vi "Server.vi"(7 "Server Alias":string, 10 "Ports":T2={"KA Port (9007)"=9007, "LtoP Port (9008)"=9008, "PtoL Port (9009)"=9009}, 11 "Local IP Address for LabVIEW Server":string="localhost") -> ()   [LabVIEW 2013, in "TS.lvlib"]
doc: "This VI does the actual TCP/IP connection with the Python side. It has three communication loops: Keep-Alive, LabVIEW-to-Python, and Python-to-LabVIEW. There's also an internal keep-alive loop, where the server has to be \"petted\" every so often, or it shuts down. This server is called dynamically so as to disconnect it from the user's framework."
uses:
  TS.lvlib
  LabVIEW Example/Supporting Code/Script Running.ctl
  LabVIEW Python Connector Message.ctl
  Ports - Keep-Alive, LabVIEW-to-Python, Python-to-LabVIEW.ctl
panel:
  out "PtoL Message":T1={"Command"="zxcvbnm,", "Data"=["asdfghjk", "qwertyui"], "Script ID"=0, "LabVIEW Server ID"="zxcvbnm,", "Python Message ID"=0}
  out "LtoP Iteration Inner":i32
  out "python response":T1={"Command"="zxcvbnm,", "Data"=["asdfghjk", "qwertyui"], "Script ID"=0, "LabVIEW Server ID"="zxcvbnm,", "Python Message ID"=0}
  out "KA Iteration":i32
  out "LtoP Messages":i32
  out "PtoL Messages":i32
  out "KA Timeout":dbl
  out "KA Messages":i32
  out "KA Message":T1={"Command"="", "Data"=[], "Script ID"=0, "LabVIEW Server ID"="zxcvbnm,", "Python Message ID"=0}
  out "LtoP Sent Message":T1={"Command"="zxcvbnm,", "Data"=["asdfghjk", "qwertyui"], "Script ID"=0, "LabVIEW Server ID"="zxcvbnm,", "Python Message ID"=0}
  out "LtoP Iteration Outer":i32
  out "LtoP Last Error":errorcluster
  out "LtoP Last Error Timestamp":timestamp
  out "LtoP length":i32
  out "LtoP Recreating":bool
  out "PtoL Iteration":i32
  out "PtoL Last Error":errorcluster
  out "PtoL Last Error Timestamp":timestamp
  out "PtoL length":i32
  out "PtoL Recreating":bool
  out "Writer Error":errorcluster
  out "Keep-Alive Last Error Timestamp":timestamp
  out "KA length":i32
  out "Keep-Alive Recreating":bool
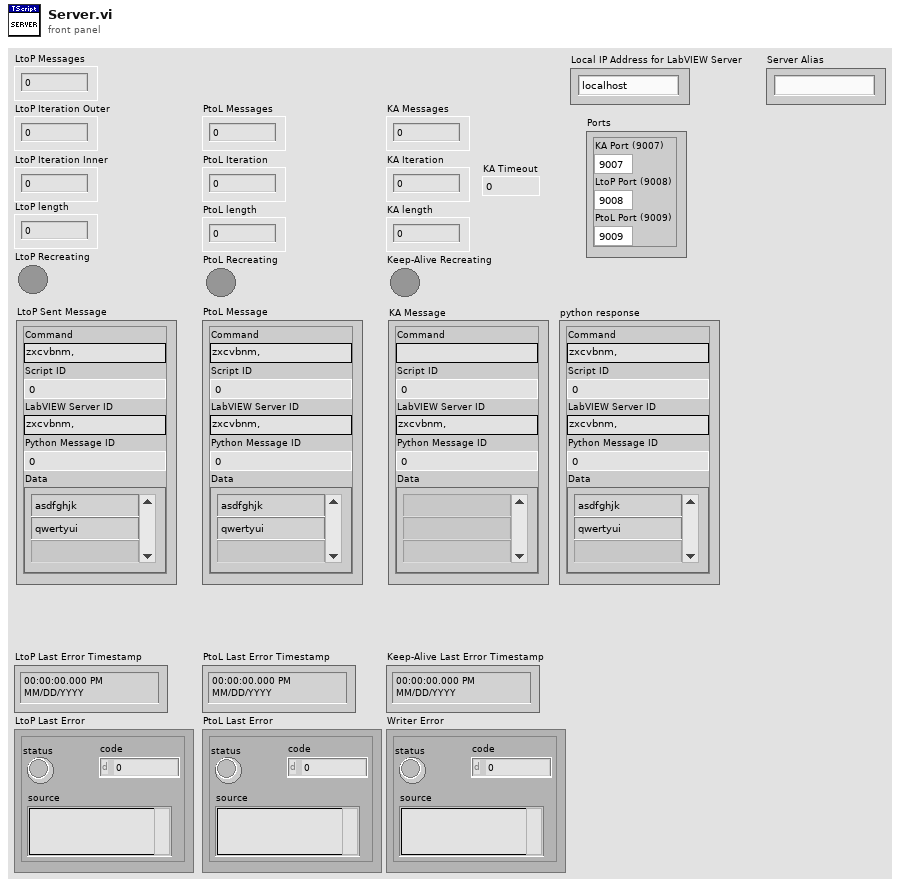
[diagram p1: front panel]
types:
  T1 = typedef "TS.lvlib/LabVIEW Python Connector Message.ctl" = cluster{"Command":string, "Data":string[], "Script ID":i64, "LabVIEW Server ID":string, "Python Message ID":i32}
  T2 = typedef "TS.lvlib/Ports - Keep-Alive, LabVIEW-to-Python, Python-to-LabVIEW.ctl" = cluster{"KA Port (9007)":u16, "LtoP Port (9008)":u16, "PtoL Port (9009)":u16}
  T3 = typedef "TS.lvlib/Script Running.ctl" = cluster{"Script ID":i64, "Script Running?":bool}
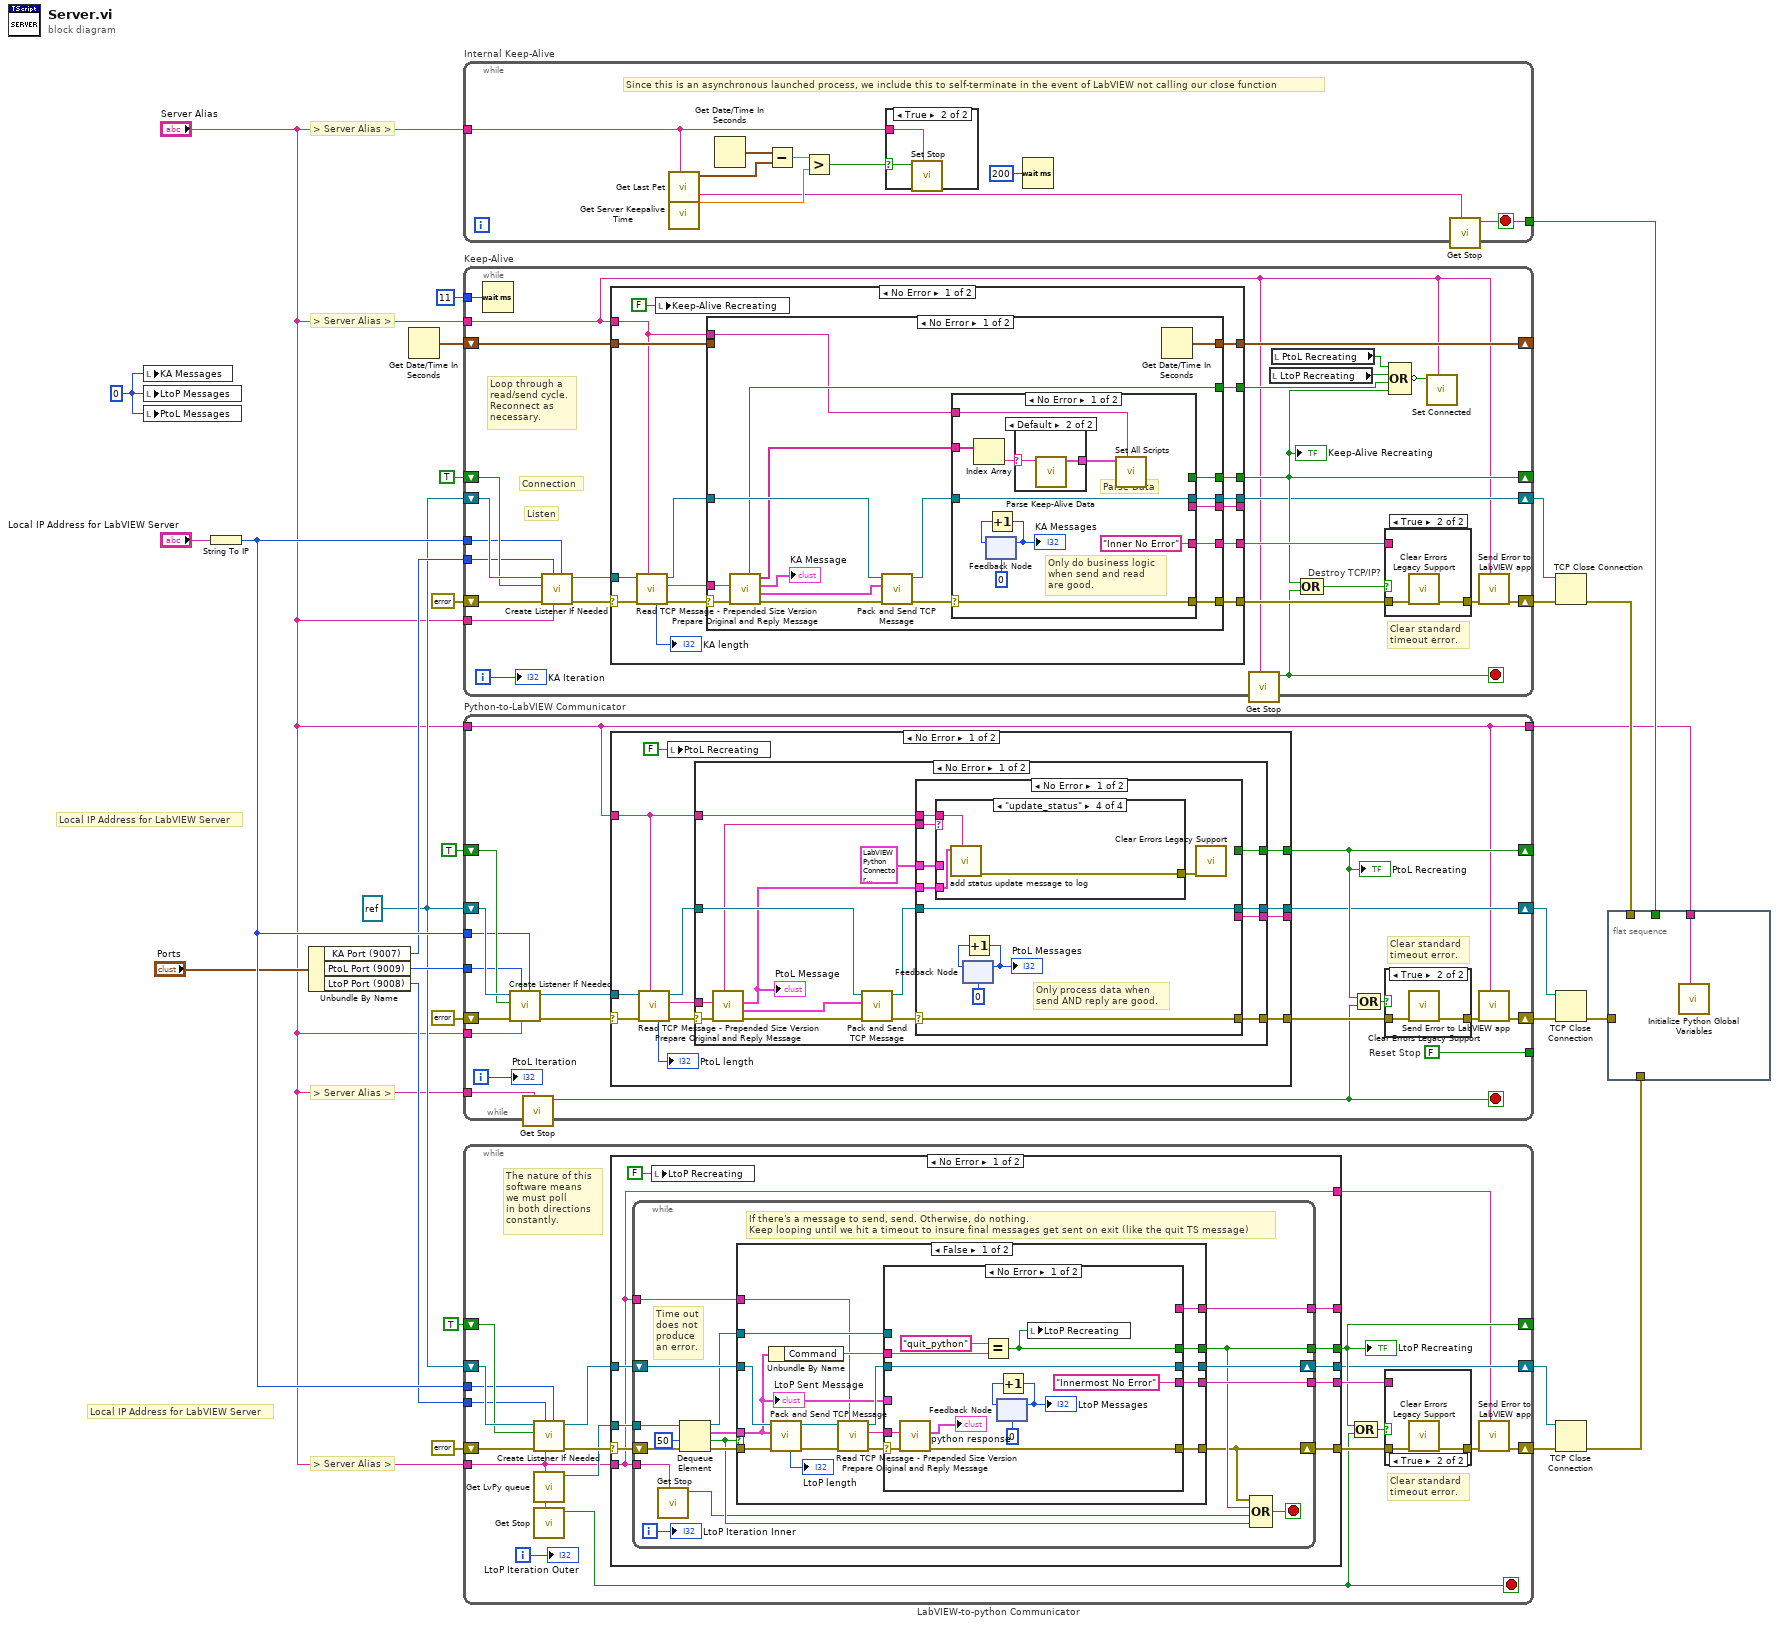
[diagram p0: block diagram]
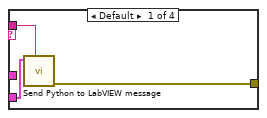
[diagram p2: hidden frame]
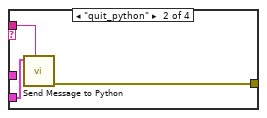
[diagram p3: hidden frame]
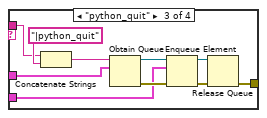
[diagram p4: hidden frame]
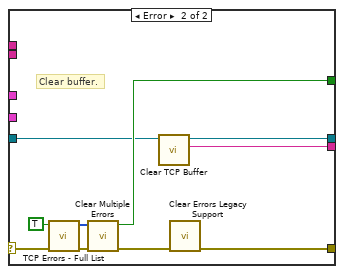
[diagram p5: hidden frame]
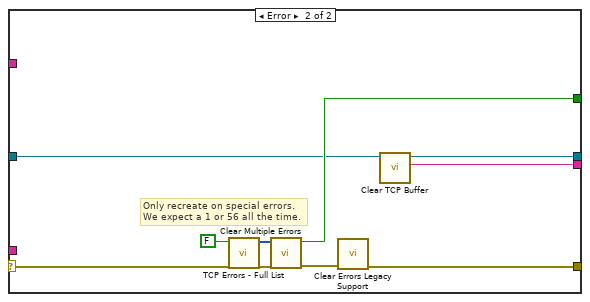
[diagram p6: hidden frame]
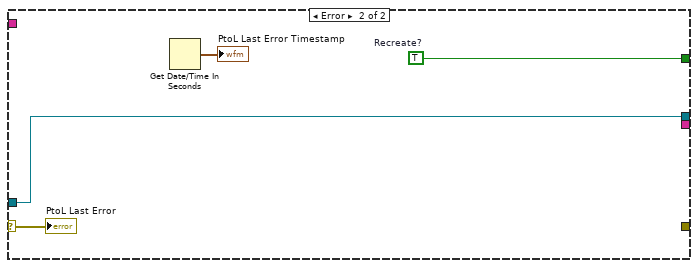
[diagram p7: hidden frame]
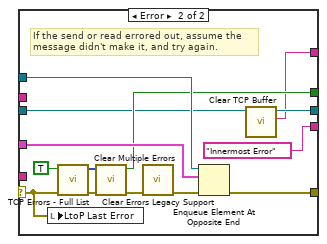
[diagram p9: hidden frame]
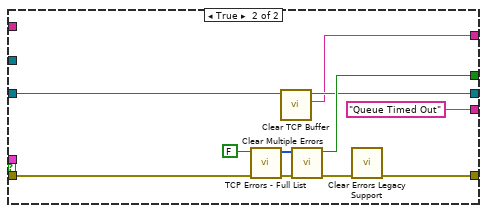
[diagram p10: hidden frame]
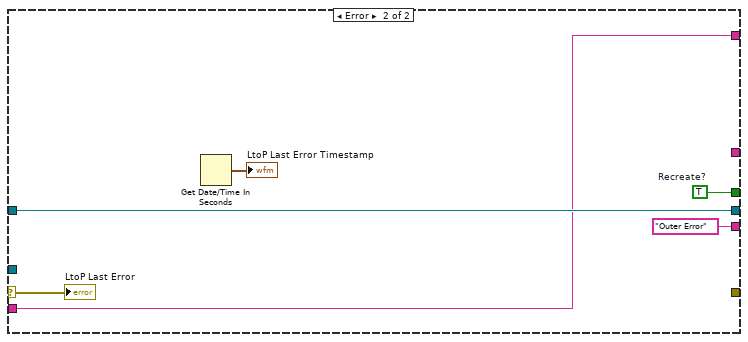
[diagram p11: hidden frame]
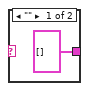
[diagram p13: hidden frame]
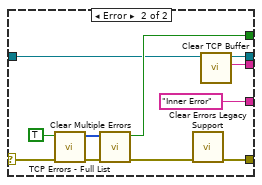
[diagram p14: hidden frame]
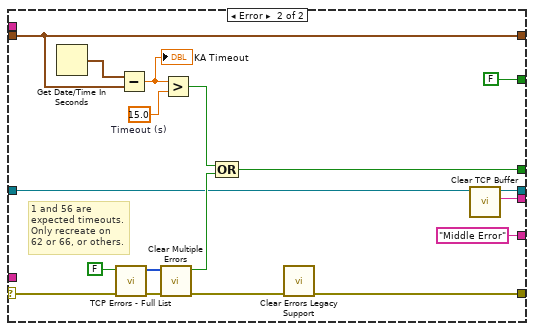
[diagram p15: hidden frame]
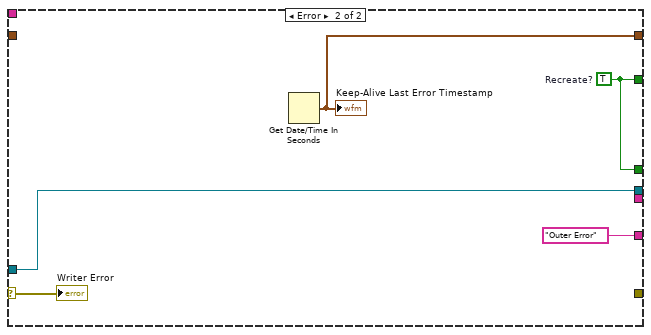
[diagram p16: hidden frame]
diagram:
  w3 = refnum<k5> refnum ("TCP Network Connection out")
  w24 = 0 ("KA Messages")
  # "> Server Alias >"
  # "> Server Alias >"
  # "> Server Alias >"
  # "> Server Alias >"
  # "Local IP Address for LabVIEW Server"
  # "Local IP Address for LabVIEW Server"
  n1 = local write "KA Messages"(w24) -> ()
  n2 = local write "LtoP Messages"(w24) -> ()
  n3 = local write "PtoL Messages"(w24) -> ()
  n4 = String To IP(1:"Local IP Address for LabVIEW Server") -> (0:w22:u32)
  n5 = Unbundle By Name("Ports") -> ("KA Port (9007)"=w18:u16, "PtoL Port (9009)"=w19:u16, "LtoP Port (9008)"=w17:u16)
  n6 = Get Date/Time In Seconds() -> (seconds since 1Jan1904=w7:timestamp)
  n7 = while "Internal Keep-Alive" {
    tunnel: [w30] -> w21
    tunnel: "Server Alias" -> [w29]
    stop <- w30 stop-if-true
    # "Since this is an asynchronous launched process, we include this to self-terminate in the event of LabVIEW not calling our close function"
    n8 = call "Get Last Pet.vi"("Server Alias"=w29) -> ("Last Pet"=w32:timestamp)  [unwired: 9 in, 1 out]
    n9 = call "Get Server Keepalive Time.vi"("Server Alias"=w29) -> ("Server Keepalive Time"=w31:dbl)  [unwired: 9 in, 1 out]
    n10 = Get Date/Time In Seconds() -> (seconds since 1Jan1904=w35:timestamp)
    n11 = Subtract(x=w35, y=w32) -> (x-y=w34:dbl)
    n12 = Greater?(x=w34, y=w31) -> (0:w33:bool)
    n13 = case shown="True" w33 {
      selector: w33 -> [_ w38]
      tunnel: w29 -> [_ w37]
      frame False {
      }
      frame True {
        n14 = call "Set Stop.vi"("Server Alias"=w37, "Stop"=w38) -> ()  [unwired: 9 in, 1 out]
      }
    }
    n15 = Wait (ms)(milliseconds to wait=u32 200) -> ()  [unwired: 1 out]
    n16 = call "Get Stop.vi"("Server Alias"=w29) -> ("Stop"=w30:bool)  [unwired: 9 in, 1 out]
  }
  n17 = while "Keep-Alive" {
    shift-right: [w52] -> w16
    shift-left: errorcluster {"status"=FALSE, "code"=0, "source"=""} ("error out") -> [w60]
    tunnel: u32 11 ("milliseconds to wait") -> [w63]
    shift-right: [w45] -> _
    shift-left: TRUE ("Recreate?") -> [w56]
    shift-right: [w43] -> w15
    shift-left: w3 -> [w59]
    tunnel: w18 -> [w54]
    shift-right: [w51] -> _
    shift-left: w7 -> [w50]
    tunnel: w22 -> [w48]
    tunnel: "Server Alias" -> [w39]
    tunnel: "Server Alias" -> [w40]
    i -> [w49]
    stop <- w41 stop-if-true
    # "Clear standard \ntimeout error."
    # "Connection"
    # "Listen"
    # "Loop through a \nread/send cycle. \nReconnect as \nnecessary."
    n18 = Wait (ms)(milliseconds to wait=w63) -> ()  [unwired: 1 out]
    n19 = call "Create Listener If Needed.vi"("net address"=w48, "Server Alias"=w40, "Port"=w54, "error in (no error)"=w60, "Recreate?"=w56, "TCP Network Connection in"=w59) -> ("error out"=w57:errorcluster, "TCP Network Connection out"=w58:refnum<k5>)  [unwired: 4 in]
    n20 = case shown="No Error" w57 {
      selector: w57 -> [w75 w141]
      tunnel: [w72 _] -> w62
      tunnel: w58 -> [w76 w140]
      tunnel: [w74 w137] -> w45
      tunnel: [w73 w140] -> w43
      tunnel: [w71 "Outer Error"] -> w55
      tunnel: [w70 w138] -> w51
      tunnel: w50 -> [w69 _]
      tunnel: [w67 w137] -> w44
      tunnel: [w66 _] -> _
      tunnel: w39 -> [w64 _]
      frame No Error {
        n21 = call "Read TCP Message - Prepended Size Version.vi"("Server Alias"=w64, "Error In"=w75, "TCP Connection In"=w76) -> ("Error Out"=w79:errorcluster, "Data Read"=w78:string, "TCP Connection Out"=w77:refnum<k5>, "Message Length"=→"KA length":i32)  [unwired: 5 in]
        n22 = local write "Keep-Alive Recreating"(FALSE ("Keep-Alive Recreating")) -> ()
        n23 = case shown="No Error" w79 {
          selector: w79 -> [w88 w127]
          tunnel: w78 -> [w86 _]
          tunnel: [w94 w136] -> w72
          tunnel: w77 -> [w91 w122]
          tunnel: [w92 w129] -> w74
          tunnel: [w93 w121] -> w73
          tunnel: [w90 "Middle Error"] -> w71
          tunnel: [w89 w131] -> w70
          tunnel: w69 -> [_ w131]
          tunnel: [w82 FALSE] -> w67
          tunnel: [w81 w120] -> w66
          tunnel: w64 -> [w80 _]
          frame No Error {
            n24 = call "Prepare Original and Reply Message.vi"("Error In"=w88, "Data Read"=w86) -> ("Error Out"=w87:errorcluster, "Reply Message"=w85:T1, "Original Message"=→"KA Message":T1, "Data Payload"=w83:string[], "\"True\" in Command?"=w82:bool)  [unwired: 4 in, 1 out]
            n25 = call "Pack and Send TCP Message.vi"("error in (no error)"=w87, "Tcp Message"=w85, "TCP Network Connection in"=w91) -> ("error out"=w95:errorcluster, "TCP Network Connection out"=w96:refnum<k5>)  [unwired: 6 in, 1 out]
            n26 = case shown="No Error" w95 {
              selector: w95 -> [w106 w118]
              tunnel: [w106 w119] -> w94
              tunnel: w96 -> [w105 w112]
              tunnel: [w105 w111] -> w93
              tunnel: [_ w116] -> w92
              tunnel: ["Inner No Error" "Inner Error"] -> w90
              tunnel: w83 -> [w102 _]
              tunnel: [_ w110] -> w81
              tunnel: w80 -> [w97 _]
              frame No Error {
                # "Only do business logic\nwhen send and read \nare good."
                # "Parse Data"
                n27 = Index Array(array=w102) -> (element=w103:string)  [unwired: 1 in]
                n28 = feedback #1(0 ("KA Messages")) -> (w100:i32)
                n29 = Increment(x=w100) -> (x+1=w101:i32)
                "KA Messages" <- w101
                n30 = feedback-in #1(w101) -> ()
                n31 = case shown="Default" w103 {
                  selector: w103 -> [_ w108]
                  tunnel: [T3[] [] ("All Scripts") w109] -> w98
                  frame "" {
                  }
                  frame Default {
                    n32 = call "Parse Keep-Alive Data.vi"("Keep-Alive Data"=w108) -> ("All Scripts"=w109:T3[])  [unwired: 10 in]
                  }
                }
                n33 = call "Set All Scripts.vi"("Server Alias"=w97, "All Scripts"=w98) -> ()  [unwired: 9 in, 1 out]
              }
              frame Error {
                n34 = call "TCP Errors - Full List.vi"("Include Expected Timeouts?"=TRUE) -> ("TCP Errors to Clear"=w115:i32[])  [unwired: 10 in]
                n35 = call "Clear Multiple Errors.vi"("Error In"=w118, "Errors to Clear"=w115) -> ("Error Out"=w113:errorcluster, "Specific Errors Cleared?"=w116:bool)  [unwired: 8 in]
                n36 = call "Clear Errors Legacy Support.vi"("error in (no error)"=w113) -> ("error out"=w119:errorcluster)  [unwired: 5 in, 1 out]
                n37 = call "Clear TCP Buffer.vi"("TCP Connection In"=w112) -> ("data out"=w110:string, "TCP Connection Out"=w111:refnum<k5>)  [unwired: 9 in]
              }
            }
            n38 = Get Date/Time In Seconds() -> (seconds since 1Jan1904=w89:timestamp)
          }
          frame Error {
            w133 = 15.0  # Timeout (s)
            # "1 and 56 are\nexpected timeouts.\nOnly recreate on\n62 or 66, or others."
            n39 = Get Date/Time In Seconds() -> (seconds since 1Jan1904=w134:timestamp)
            n40 = call "TCP Errors - Full List.vi"("Include Expected Timeouts?"=FALSE) -> ("TCP Errors to Clear"=w123:i32[])  [unwired: 10 in]
            n41 = Subtract(x=w134, y=w131) -> (x-y=w132:dbl)
            "KA Timeout" <- w132
            n42 = call "Clear Multiple Errors.vi"("Error In"=w127, "Errors to Clear"=w123) -> ("Error Out"=w126:errorcluster, "Specific Errors Cleared?"=w125:bool)  [unwired: 8 in]
            n43 = Greater?(x=w132, y=w133) -> (0:w130:bool)
            n44 = Compound Arithmetic op=OR(w130, w125) -> (w129:bool)
            n45 = call "Clear Errors Legacy Support.vi"("error in (no error)"=w126) -> ("error out"=w136:errorcluster)  [unwired: 5 in, 1 out]
            n46 = call "Clear TCP Buffer.vi"("TCP Connection In"=w122) -> ("data out"=w120:string, "TCP Connection Out"=w121:refnum<k5>)  [unwired: 9 in]
          }
        }
      }
      frame Error {
        w137 = TRUE  # Recreate?
        n47 = Get Date/Time In Seconds() -> (seconds since 1Jan1904=w138:timestamp)
        "Keep-Alive Last Error Timestamp" <- w138
        "Writer Error" <- w141
      }
    }
    "Keep-Alive Recreating" <- w45
    n48 = call "Get Stop.vi"("Server Alias"=w39) -> ("Stop"=w41:bool)  [unwired: 9 in, 1 out]
    n49 = local read "LtoP Recreating"() -> (w47:bool)
    n50 = local read "PtoL Recreating"() -> (w46:bool)
    n51 = Compound Arithmetic op=OR(w45, w41) -> (w61:bool)
    n52 = case "Destroy TCP/IP?" shown="True" w61 {
      tunnel: w62 -> [w142 w143]
      tunnel: [w142 w144] -> w53
      tunnel: w55 -> [_ _]
      frame False {
      }
      frame True {
        n53 = call "Clear Errors Legacy Support.vi"("error in (no error)"=w143) -> ("error out"=w144:errorcluster)  [unwired: 5 in, 1 out]
      }
    }
    n54 = Compound Arithmetic op=OR(w46, w47, w44, w45) -> (invert w42:bool)
    n55 = call "Set Connected.vi"("Server Alias"=w39, "Connected"=w42) -> ()  [unwired: 9 in, 1 out]
    n56 = call "Send Error to LabVIEW app.vi"("Server Alias"=w39, "error in (no error)"=w53) -> ("error out"=w52:errorcluster)  [unwired: 9 in]
    "KA Iteration" <- w49
  }
  n57 = while "Python-to-LabVIEW Communicator" {
    shift-right: [w153] -> w13
    shift-left: errorcluster {"status"=FALSE, "code"=0, "source"=""} ("error out") -> [w162]
    shift-right: [w150] -> w12
    shift-left: w3 -> [w161]
    tunnel: [w163] -> _
    shift-right: [w156] -> _
    shift-left: TRUE ("Recreate?") -> [w157]
    tunnel: w19 -> [w155]
    tunnel: w22 -> [w151]
    tunnel: "Server Alias" -> [w147]
    tunnel: "Server Alias" -> [w146]
    tunnel: [w146] -> w2
    tunnel: "Server Alias" -> [w145]
    i -> [w152]
    stop <- w148 stop-if-true
    w163 = FALSE  # Reset Stop
    # "Clear standard \ntimeout error."
    n58 = call "Create Listener If Needed.vi"("net address"=w151, "Server Alias"=w145, "Port"=w155, "error in (no error)"=w162, "Recreate?"=w157, "TCP Network Connection in"=w161) -> ("error out"=w149:errorcluster, "TCP Network Connection out"=w160:refnum<k5>)  [unwired: 4 in]
    n59 = call "Get Stop.vi"("Server Alias"=w147) -> ("Stop"=w148:bool)  [unwired: 9 in, 1 out]
    n60 = case shown="No Error" w149 {
      selector: w149 -> [w172 w240]
      tunnel: w160 -> [w171 w241]
      tunnel: [w170 w241] -> w150
      tunnel: [w169 _] -> w159
      tunnel: [w168 w239] -> w156
      tunnel: [w166 _] -> _
      tunnel: w146 -> [w164 _]
      frame No Error {
        n61 = call "Read TCP Message - Prepended Size Version.vi"("Server Alias"=w164, "Error In"=w172, "TCP Connection In"=w171) -> ("Error Out"=w175:errorcluster, "Data Read"=w174:string, "TCP Connection Out"=w173:refnum<k5>, "Message Length"=→"PtoL length":i32)  [unwired: 5 in]
        n62 = local write "PtoL Recreating"(FALSE ("PtoL Recreating")) -> ()
        n63 = case shown="No Error" w175 {
          selector: w175 -> [w184 w234]
          tunnel: w174 -> [w183 _]
          tunnel: [w186 w237] -> w169
          tunnel: w173 -> [w188 w231]
          tunnel: [w187 w230] -> w170
          tunnel: [w185 w235] -> w168
          tunnel: [w178 w229] -> w166
          tunnel: w164 -> [w177 _]
          frame No Error {
            n64 = call "Prepare Original and Reply Message.vi"("Error In"=w184, "Data Read"=w183) -> ("Error Out"=w179:errorcluster, "Reply Message"=w180:T1, "Original Message"=w181:T1, "Command"=w182:string)  [unwired: 4 in, 2 out]
            "PtoL Message" <- w181
            n65 = call "Pack and Send TCP Message.vi"("error in (no error)"=w179, "Tcp Message"=w180, "TCP Network Connection in"=w188) -> ("error out"=w190:errorcluster, "TCP Network Connection out"=w189:refnum<k5>)  [unwired: 6 in, 1 out]
            n66 = case shown="No Error" w190 {
              selector: w190 -> [w200 w226]
              tunnel: [w200 w228] -> w186
              tunnel: w189 -> [w199 w222]
              tunnel: [w199 w221] -> w187
              tunnel: [_ w224] -> w185
              tunnel: w181 -> [w197 _]
              tunnel: w182 -> [w196 _]
              tunnel: [_ w220] -> w178
              tunnel: w177 -> [w192 _]
              tunnel: T1 {"Command"="zxcvbnm,", "Data"=["asdfghjk", "qwertyui"], "Script ID"=0, "LabVIEW Server ID"="zxcvbnm,", "Python Message ID"=0} -> [w191 _]
              frame No Error {
                # "Only process data when\nsend AND reply are good."
                n67 = case shown="\"update_status\"" w196 {
                  tunnel: w197 -> [w203 w206 w213 w219]
                  tunnel: [w202 w205 w211 w218] -> w198
                  tunnel: w192 -> [w201 w204 w207 w217]
                  tunnel: w191 -> [_ _ w209 _]
                  frame Default {
                    n68 = call "Send Python to LabVIEW message.vi"("Server Alias"=w201, "Message"=w203) -> ("error out"=w202:errorcluster)  [unwired: 9 in]
                  }
                  frame "quit_python" {
                    n69 = call "Send Message to Python.vi"("Server Alias"=w204, "Message"=w206) -> ("error out"=w205:errorcluster)  [unwired: 9 in]
                  }
                  frame "python_quit" {
                    n70 = Concatenate Strings(w207, "|python_quit" ("name (unnamed)")) -> (w208:string)
                    n71 = Obtain Queue(name (unnamed)=w208, element data type=w209) -> (queue out=w216:refnum<queue>, error out=w215:errorcluster)  [unwired: 3 in, 1 out]
                    n72 = Enqueue Element(queue=w216, element=w213, error in (no error)=w215) -> (queue out=w210:refnum<queue>, error out=w212:errorcluster)  [unwired: 1 in, 1 out]
                    n73 = Release Queue(queue=w210, error in (no error)=w212) -> (error out=w211:errorcluster)  [unwired: 1 in, 2 out]
                  }
                  frame "update_status" {
                    n74 = call "add status update message to log.vi"("Server Alias"=w217, "Tcp Message"=w219) -> ("Error Out"=w218:errorcluster)  [unwired: 9 in]
                  }
                }
                n75 = feedback #2(0 ("KA Messages")) -> (w194:i32)
                n76 = Increment(x=w194) -> (x+1=w193:i32)
                "PtoL Messages" <- w193
                n77 = feedback-in #2(w193) -> ()
                n78 = call "Clear Errors Legacy Support.vi"("error in (no error)"=w198) -> ()  [unwired: 5 in, 2 out]
              }
              frame Error {
                # "Clear buffer."
                n79 = call "TCP Errors - Full List.vi"("Include Expected Timeouts?"=TRUE) -> ("TCP Errors to Clear"=w227:i32[])  [unwired: 10 in]
                n80 = call "Clear Multiple Errors.vi"("Error In"=w226, "Errors to Clear"=w227) -> ("Error Out"=w225:errorcluster, "Specific Errors Cleared?"=w224:bool)  [unwired: 8 in]
                n81 = call "Clear TCP Buffer.vi"("TCP Connection In"=w222) -> ("data out"=w220:string, "TCP Connection Out"=w221:refnum<k5>)  [unwired: 9 in]
                n82 = call "Clear Errors Legacy Support.vi"("error in (no error)"=w225) -> ("error out"=w228:errorcluster)  [unwired: 5 in, 1 out]
              }
            }
          }
          frame Error {
            # "Only recreate on special errors.\nWe expect a 1 or 56 all the time."
            n83 = call "TCP Errors - Full List.vi"("Include Expected Timeouts?"=FALSE) -> ("TCP Errors to Clear"=w232:i32[])  [unwired: 10 in]
            n84 = call "Clear Multiple Errors.vi"("Error In"=w234, "Errors to Clear"=w232) -> ("Error Out"=w236:errorcluster, "Specific Errors Cleared?"=w235:bool)  [unwired: 8 in]
            n85 = call "Clear Errors Legacy Support.vi"("error in (no error)"=w236) -> ("error out"=w237:errorcluster)  [unwired: 5 in, 1 out]
            n86 = call "Clear TCP Buffer.vi"("TCP Connection In"=w231) -> ("data out"=w229:string, "TCP Connection Out"=w230:refnum<k5>)  [unwired: 9 in]
          }
        }
      }
      frame Error {
        w239 = TRUE  # Recreate?
        n87 = Get Date/Time In Seconds() -> (seconds since 1Jan1904=→"PtoL Last Error Timestamp":timestamp)
        "PtoL Last Error" <- w240
      }
    }
    "PtoL Recreating" <- w156
    n88 = Compound Arithmetic op=OR(w156, w148) -> (w158:bool)
    n89 = case shown="True" w158 {
      tunnel: [w242 w244] -> w154
      tunnel: w159 -> [w242 w243]
      frame False {
      }
      frame True {
        n90 = call "Clear Errors Legacy Support.vi"("error in (no error)"=w243) -> ("error out"=w244:errorcluster)  [unwired: 5 in, 1 out]
      }
    }
    n91 = call "Send Error to LabVIEW app.vi"("Server Alias"=w146, "error in (no error)"=w154) -> ("error out"=w153:errorcluster)  [unwired: 9 in]
    "PtoL Iteration" <- w152
  }
  n92 = while "LabVIEW-to-python Communicator" {
    shift-right: [w252] -> w10
    shift-left: errorcluster {"status"=FALSE, "code"=0, "source"=""} ("error out") -> [w262]
    shift-right: [w249] -> w9
    shift-left: w3 -> [w260]
    shift-right: [w255] -> _
    shift-left: TRUE -> [w257]
    tunnel: w17 -> [w254]
    tunnel: w22 -> [w250]
    tunnel: "Server Alias" -> [w246]
    i -> [w251]
    stop <- w247 stop-if-true
    # "Clear standard \ntimeout error."
    # "The nature of this \nsoftware means \nwe must poll\nin both directions \nconstantly."
    n93 = call "Create Listener If Needed.vi"("net address"=w250, "Server Alias"=w246, "Port"=w254, "error in (no error)"=w262, "Recreate?"=w257, "TCP Network Connection in"=w260) -> ("error out"=w261:errorcluster, "TCP Network Connection out"=w259:refnum<k5>)  [unwired: 4 in]
    n94 = call "Get LvPy queue.vi"("Server Alias"=w246) -> ("LvPy queue"=w248:refnum<queue>)  [unwired: 9 in, 1 out]
    n95 = call "Get Stop.vi"("Server Alias"=w246) -> ("Stop"=w247:bool)  [unwired: 9 in, 1 out]
    n96 = case shown="No Error" w261 {
      selector: w261 -> [w271 w348]
      tunnel: [w273 w349] -> w249
      tunnel: w259 -> [w270 w349]
      tunnel: [w272 _] -> w263
      tunnel: [w269 "Outer Error"] -> w256
      tunnel: [w268 w346] -> w255
      tunnel: w248 -> [w267 _]
      tunnel: [w266 _] -> _
      tunnel: w246 -> [w264 w344]
      tunnel: [w264 w344] -> w245
      frame No Error {
        n97 = while {
          tunnel: [w285] -> w269
          tunnel: [w281] -> w268
          tunnel: w267 -> [w284]
          shift-right: [w280] -> w272
          shift-left: w271 -> [w289]
          shift-right: [w291] -> w273
          shift-left: w270 -> [w287]
          tunnel: [w277] -> w266
          tunnel: w264 -> [w276]
          tunnel: w264 -> [w274]
          i -> [w278]
          stop <- w283 stop-if-true
          # "Time out\ndoes not\nproduce\nan error."
          # "If there's a message to send, send. Otherwise, do nothing.\nKeep looping until we hit a timeout to insure final messages get sent on exit (like the quit TS message)"
          n98 = call "Get Stop.vi"("Server Alias"=w276) -> ("Stop"=w275:bool)  [unwired: 9 in, 1 out]
          n99 = Dequeue Element(queue=w284, timeout in ms (-1)=50, error in (no error)=w289) -> (queue out=w279:refnum<queue>, element=w288:T1, timed out?=w282:bool, error out=w286:errorcluster)
          n100 = case shown="False" w282 {
            tunnel: [w304 w343] -> w280
            tunnel: w287 -> [w303 w337]
            tunnel: [w305 w336] -> w291
            tunnel: w288 -> [w296 _]
            tunnel: w286 -> [w301 w335]
            tunnel: [w300 "Queue Timed Out"] -> w285
            tunnel: [w299 w340] -> w281
            tunnel: w279 -> [w295 _]
            tunnel: [w293 w334] -> w277
            tunnel: w274 -> [w292 _]
            frame False {
              n101 = Unbundle By Name(w296) -> ("Command"=w297:string)
              n102 = call "Pack and Send TCP Message.vi"("error in (no error)"=w301, "Tcp Message"=w296, "TCP Network Connection in"=w303) -> ("error out"=w294:errorcluster, "TCP Network Connection out"=w302:refnum<k5>, "Message Length"=→"LtoP length":i32)  [unwired: 6 in]
              n103 = call "Read TCP Message - Prepended Size Version.vi"("Server Alias"=w292, "Error In"=w294, "TCP Connection In"=w302) -> ("Error Out"=w306:errorcluster, "Data Read"=w307:string, "TCP Connection Out"=w308:refnum<k5>)  [unwired: 5 in, 1 out]
              n104 = case shown="No Error" w306 {
                selector: w306 -> [w315 w329]
                tunnel: w307 -> [w314 _]
                tunnel: [w312 w330] -> w304
                tunnel: w308 -> [w320 w323]
                tunnel: [w320 w322] -> w305
                tunnel: ["Innermost No Error" "Innermost Error"] -> w300
                tunnel: [w316 w327] -> w299
                tunnel: w297 -> [w318 _]
                tunnel: w296 -> [_ w331]
                tunnel: w295 -> [_ w332]
                tunnel: [_ w321] -> w293
                frame No Error {
                  n105 = call "Prepare Original and Reply Message.vi"("Error In"=w315, "Data Read"=w314) -> ("Error Out"=w312:errorcluster, "Original Message"=→"python response":T1)  [unwired: 4 in, 4 out]
                  n106 = Equal?(x="quit_python", y=w318) -> (x = y?=w316:bool)
                  n107 = feedback #3(0 ("KA Messages")) -> (w310:i32)
                  n108 = Increment(x=w310) -> (x+1=w311:i32)
                  "LtoP Messages" <- w311
                  n109 = feedback-in #3(w311) -> ()
                  n110 = local write "LtoP Recreating"(w316) -> ()
                }
                frame Error {
                  # "If the send or read errored out, assume the \nmessage didn't make it, and try again."
                  n111 = local write "LtoP Last Error"(w329) -> ()
                  n112 = call "TCP Errors - Full List.vi"("Include Expected Timeouts?"=TRUE) -> ("TCP Errors to Clear"=w328:i32[])  [unwired: 10 in]
                  n113 = call "Clear Multiple Errors.vi"("Error In"=w329, "Errors to Clear"=w328) -> ("Error Out"=w326:errorcluster, "Specific Errors Cleared?"=w327:bool)  [unwired: 8 in]
                  n114 = call "Clear Errors Legacy Support.vi"("error in (no error)"=w326) -> ("error out"=w325:errorcluster)  [unwired: 5 in, 1 out]
                  n115 = Enqueue Element At Opposite End(queue=w332, element=w331, error in (no error)=w325) -> (error out=w330:errorcluster)  [unwired: 1 in, 2 out]
                  n116 = call "Clear TCP Buffer.vi"("TCP Connection In"=w323) -> ("data out"=w321:string, "TCP Connection Out"=w322:refnum<k5>)  [unwired: 9 in]
                }
              }
              "LtoP Sent Message" <- w296
            }
            frame True {
              n117 = call "TCP Errors - Full List.vi"("Include Expected Timeouts?"=FALSE) -> ("TCP Errors to Clear"=w338:i32[])  [unwired: 10 in]
              n118 = call "Clear TCP Buffer.vi"("TCP Connection In"=w337) -> ("data out"=w334:string, "TCP Connection Out"=w336:refnum<k5>)  [unwired: 9 in]
              n119 = call "Clear Multiple Errors.vi"("Error In"=w335, "Errors to Clear"=w338) -> ("Error Out"=w341:errorcluster, "Specific Errors Cleared?"=w340:bool)  [unwired: 8 in]
              n120 = call "Clear Errors Legacy Support.vi"("error in (no error)"=w341) -> ("error out"=w343:errorcluster)  [unwired: 5 in, 1 out]
            }
          }
          n121 = Compound Arithmetic op=OR(w280, w281, w275, w282) -> (w283:bool)
          "LtoP Iteration Inner" <- w278
        }
        n122 = local write "LtoP Recreating"(FALSE ("LtoP Recreating")) -> ()
      }
      frame Error {
        w346 = TRUE  # Recreate?
        n123 = Get Date/Time In Seconds() -> (seconds since 1Jan1904=→"LtoP Last Error Timestamp":timestamp)
        "LtoP Last Error" <- w348
      }
    }
    "LtoP Recreating" <- w255
    n124 = Compound Arithmetic op=OR(w255, w247) -> (w258:bool)
    n125 = case shown="True" w258 {
      tunnel: w263 -> [w350 w351]
      tunnel: [w350 w352] -> w253
      tunnel: w256 -> [_ _]
      frame False {
      }
      frame True {
        n126 = call "Clear Errors Legacy Support.vi"("error in (no error)"=w351) -> ("error out"=w352:errorcluster)  [unwired: 5 in, 1 out]
      }
    }
    n127 = call "Send Error to LabVIEW app.vi"("Server Alias"=w245, "error in (no error)"=w253) -> ("error out"=w252:errorcluster)  [unwired: 9 in]
    "LtoP Iteration Outer" <- w251
  }
  n128 = TCP Close Connection(connection ID=w15, error in (no error)=w16) -> (error out=w14:errorcluster)  [unwired: 1 in, 1 out]
  n129 = TCP Close Connection(connection ID=w12, error in (no error)=w13) -> (error out=w11:errorcluster)  [unwired: 1 in, 1 out]
  n130 = TCP Close Connection(connection ID=w9, error in (no error)=w10) -> (error out=w8:errorcluster)  [unwired: 1 in, 1 out]
  n131 = flat-sequence {
    tunnel: w8 -> [_]
    tunnel: w14 -> [_]
    tunnel: w21 -> [_]
    tunnel: w11 -> [_]
    tunnel: w2 -> [w353]
    frame #0 {
      n132 = call "Initialize Python Global Variables.vi"("Server Alias"=w353) -> ()  [unwired: 10 in, 1 out]
    }
  }
